vi "SVT Weighting Filter (1 Ch).vi"(5 "reset filter (F)":bool, 7 "error in (no error)":errorcluster, 9 "weighting":u16(ring) items=["Linear", "A-weighting", "B-weighting", "C-weighting"], 10 "scaled signal [EU]":waveform(dbl)) -> (0 "error out":errorcluster, 3 "weighted signal [EU]":waveform(dbl))   [LabVIEW 2017, in "SoundVib_ABCWeighting.lvlib"]
doc: "Applies the selected weighting to <B>scaled signal [EU]</B>. This VI complies with ANSI S1.4-1983, ANSI S1.42-2001, IEC 61672-1:2002, and JIS C 1509-1:2005 standards. Use Each instance of this VI maintains its own state; use the N Channel instance of this VI to process an array of channels. This VI operates on time-continuous data; it resets on a discontinuity. Wire data to the <B>scaled signal [EU]</B> input to determine the polymorphic instance to use or manually select the instance."
uses:
  <vilib>/addons/Sound and Vibration/svt_Weighting/SoundVib_ABCWeighting.lvlib
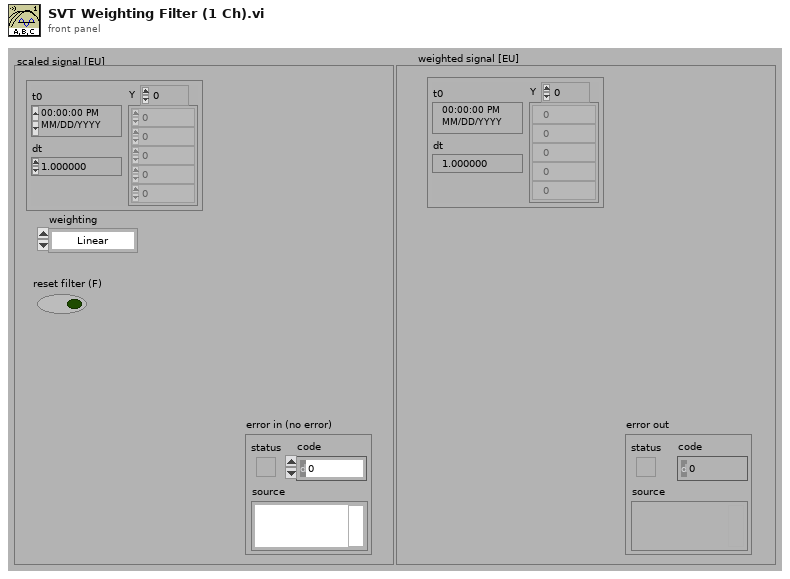
[diagram p1: front panel]
types:
  T1 = typedef "svc_Weighting Filter Text Ring.ctl" = u16
  T2 = cluster{"filter structure":enum32{"IIR 2nd Order", "IIR 4th Order"}, "Reverse Coefficients":dbl[], "Forward Coefficients":dbl[]}
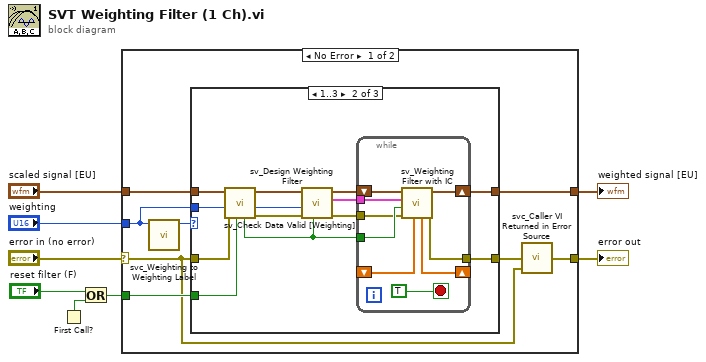
[diagram p0: block diagram]
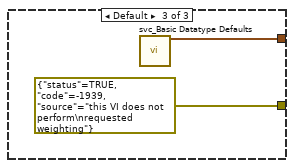
[diagram p3: hidden frame]
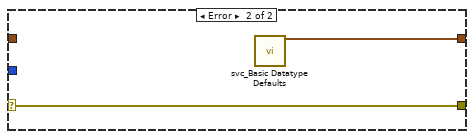
[diagram p4: hidden frame]
diagram:
  n1 = First Call?() -> (First Call?: T/F=w1:bool)
  n2 = Or(x="reset filter (F)", y=w1) -> (x .or. y?=w5:bool)
  n3 = case shown="No Error" "error in (no error)" {
    selector: "error in (no error)" -> [w9 w44]
    tunnel: [w13 w44] -> w8
    tunnel: [w16 w43] -> w7
    tunnel: "scaled signal [EU]" -> [w15 _]
    tunnel: w5 -> [w14 _]
    tunnel: "weighting" -> [w10 _]
    frame No Error {
      n4 = call <vilib>:"svc_Weighting to Weighting Label.vi"("weighting filter"=w10) -> ("weighting enum"=w11:T1)  [unwired: 9 in, 1 out]
      n5 = case shown="1..3" w11 {
        tunnel: [w17 w27 errorcluster {"status"=TRUE, "code"=-1939, "source"="this VI does not perform\nrequested weighting"} ("error out")] -> w12
        tunnel: [w18 w31 w42] -> w16
        tunnel: w15 -> [w18 w30 _]
        tunnel: w9 -> [w17 w29 _]
        tunnel: w14 -> [_ w28 _]
        tunnel: w10 -> [_ w26 _]
        frame 0 {
          # "if (weighting == Linear )\nSkip weighting()"
        }
        frame 1..3 {
          n6 = call <vilib>:"sv_Check Data Valid [Weighting].vi"("reset (in)"=w28, "error in (no error)"=w29, "weighting"=w26, "signal in [X]"=w30) -> ("error out"=w23:errorcluster, "weighting"=w24:T1, "signal out [X]"=w25:waveform(dbl), "reset (out)"=w22:bool)  [unwired: 4 in]
          n7 = call <vilib>:"sv_Design Weighting Filter.vi"("reset filter (F)"=w22, "error in (no error)"=w23, "weighting"=w24, "scaled signal"=w25) -> ("error out"=w19:errorcluster, "filter coefficients"=w20:T2, "dup scaled signal"=w21:waveform(dbl))  [unwired: 5 in]
          n8 = while {
            shift-left: _ -> [w37]
            shift-right: [w36] -> _
            tunnel: w22 -> [w35]
            tunnel: [w40] -> w27
            tunnel: w20 -> [w33]
            tunnel: w19 -> [w32]
            shift-right: [w39] -> w31
            shift-left: w21 -> [w34]
            stop <- TRUE stop-if-true
            n9 = call <vilib>:"sv_Weighting Filter with IC.vi"("Initial Filter State"=w37, "error in (no error)"=w32, "reset filter (F)"=w35, "filter coefficients"=w33, "signal [V]"=w34) -> ("error out"=w40:errorcluster, "filtered signal [EU]"=w39:waveform(dbl), "Final Filter State"=w36:dbl[])  [unwired: 4 in]
          }
        }
        frame Default {
          n10 = call <vilib>:"svc_Basic Datatype Defaults.vi"() -> ("empty waveform"=w42:waveform(dbl))  [unwired: 7 in, 12 out]
        }
      }
      n11 = call <vilib>:"svc_Caller VI Returned in Error Source.vi"("warning input to caller"=w9, "error in (no error)"=w12) -> ("error out"=w13:errorcluster)  [unwired: 3 in]
    }
    frame Error {
      n12 = call <vilib>:"svc_Basic Datatype Defaults.vi"() -> ("empty waveform"=w43:waveform(dbl))  [unwired: 7 in, 12 out]
    }
  }
  "error out" <- w8
  "weighted signal [EU]" <- w7
